vi "Write Command.vi"(8 "error in (no error)":errorcluster, 10 "Message":refnum<class "Message Interface.lvclass">, 11 "Websocket Client Handler in":refnum<class "Websocket Client Handler.lvclass">) -> (0 "error out":errorcluster, 3 "Websocket Client Handler out":refnum<class "Websocket Client Handler.lvclass">)   [LabVIEW 2016, in "Stream Mediator.lvlib" / "Websocket Client Handler.lvclass"]
doc: "--\nCopyright © 2017 Composed SystemsI All rights reserved.\n\nAuthor: Jon McBee <jon.mcbee@composed.io>\n\nThis library is provided \"AS IS\" ,WITHOUT WARRANTIES OR\nCONDITIONS OF ANY KIND, either express or implied.\n\nComposed Systems -- composed.io\n\nStream 0.0.1.1\nJon McBee - Composed Systems\nCopyright (c) 2017, Composed Systems"
uses:
  <userlib>/Composed Systems/Stream/Mediator/Classes/Websocket Client Handler Actor/Websocket Client Handler/Websocket Client Handler.lvclass
  <userlib>/Composed Systems/Stream/Mediator/Classes/Message Interface/Message Interface.lvclass
  <userlib>/Composed Systems/Stream/Mediator/Classes/Websocket Client Handler Actor/Websocket Client Handler/Websocket Client Handler.lvclass/Websocket Client Handler.ctl
  <vilib>/MediaMongrels Ltd/WebSockets/WebSockets/WebSockets.lvlib
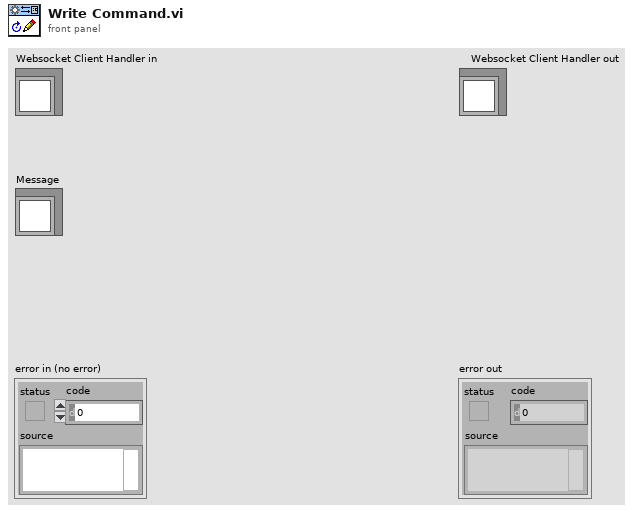
[diagram p1: front panel]
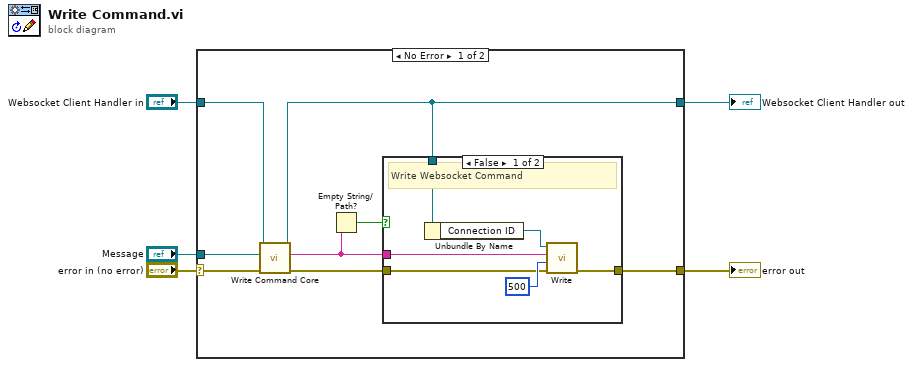
[diagram p0: block diagram]
diagram:
  n1 = case shown="No Error" "error in (no error)" {
    selector: "error in (no error)" -> [w11 w22]
    tunnel: [w13 w22] -> w4
    tunnel: [w8 w21] -> w2
    tunnel: "Websocket Client Handler in" -> [w9 w21]
    tunnel: "Message" -> [w7 _]
    frame No Error {
      n2 = call-dynamic "Write Command Core.vi"("error in (no error)"=w11, "Message"=w7, "Websocket Client Handler in"=w9) -> ("error out"=w10:errorcluster, "JSON String"=w6:string, "Websocket Client Handler out"=w8:refnum<class "Websocket Client Handler.lvclass">)  [unwired: 6 in]
      n3 = Empty String/Path?(string/path=w6) -> (empty?=w12:bool)
      n4 = case shown="False" w12 {
        tunnel: w10 -> [w18 w20]
        tunnel: [w17 w20] -> w13
        tunnel: w8 -> [w16 _]
        tunnel: w6 -> [w14 _]
        frame False {
          # "Write Websocket Command"
          n5 = Unbundle By Name(w16) -> ("Connection ID"=w15:refnum<k5>)
          n6 = call <vilib>:"Write.vi"("error in (no error)"=w18, "timeout ms (5000)"=500, "Data"=w14, "WebSocket Connection in"=w15) -> ("error out"=w17:errorcluster)  [unwired: 6 in, 1 out]
        }
        frame True {
          # "#ERROR"
          # "Empty String - Don't Write"
        }
      }
    }
    frame Error {
    }
  }
  "error out" <- w4
  "Websocket Client Handler out" <- w2
